vi "SMC.vi"(6 "e_prev":dbl, 7 "t":dbl, 8 "q":dbl, 9 "SP":dbl, 10 "a":dbl, 11 "gain":dbl) -> (2 "e_out":dbl, 3 "u":dbl)   [LabVIEW 2014]
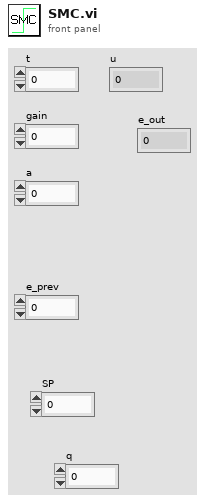
[diagram p1: front panel]
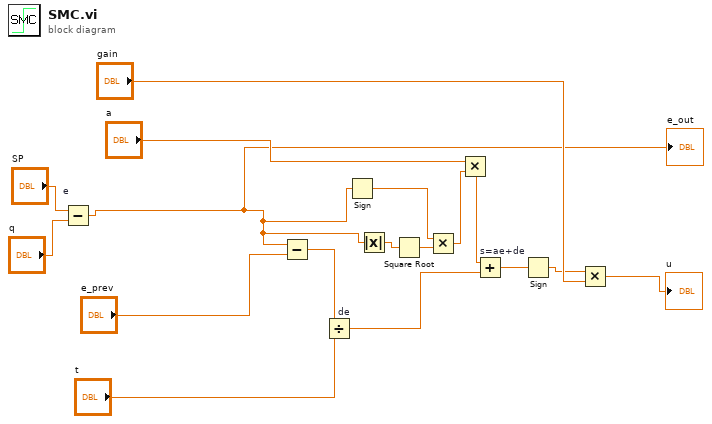
[diagram p0: block diagram]
diagram:
  n1 = Subtract "e"(x="SP", y="q") -> (x-y=w1:dbl)
  "e_out" <- w1
  n2 = Subtract(x=w1, y="e_prev") -> (x-y=w5:dbl)
  n3 = Divide "de"(x=w5, y="t") -> (x/y=w9:dbl)
  n4 = Sign(1:w1) -> (0:w16:dbl)
  n5 = Absolute Value(x=w1) -> (abs(x)=w14:dbl)
  n6 = Square Root(x=w14) -> (sqrt(x)=w15:dbl)
  n7 = Multiply(x=w16, y=w15) -> (x*y=w17:dbl)
  n8 = Multiply(x="a", y=w17) -> (x*y=w8:dbl)
  n9 = Add "s=ae+de"(x=w8, y=w9) -> (x+y=w10:dbl)
  n10 = Sign(1:w10) -> (0:w11:dbl)
  n11 = Multiply(x=w11, y="gain") -> (x*y=→"u":dbl)
